vi "Wait For Key File.vi"(8 "error in":errorcluster, 11 "key file path":path) -> (0 "error out":errorcluster)   [LabVIEW 2020, in "Measurement Plugin Discovery V1.lvlib"]
uses:
  Measurement Plugin Discovery V1.lvlib
  Measurement Plugin Measurement Server/Helpers/Error Strings Global Internal.vi
  <vilib>/ErrorRing/Error Ring.xnode
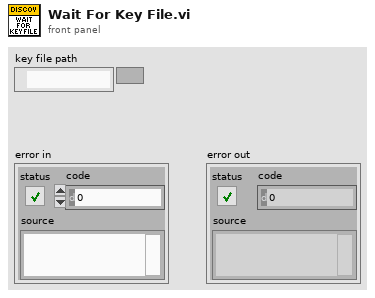
[diagram p1: front panel]
types:
  T1 = enum16{"open", "replace", "create", "open or create", "replace or create", "replace or create with confirmation"}
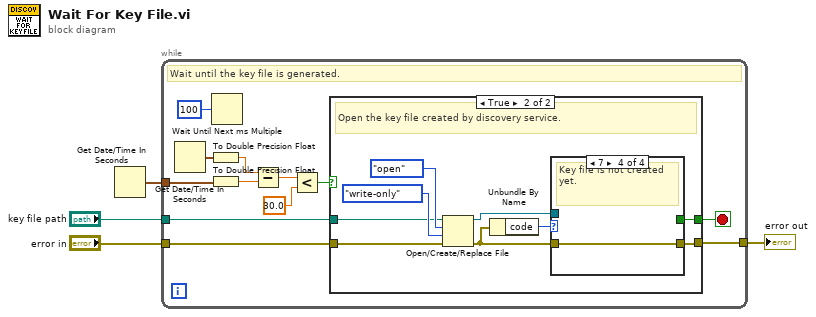
[diagram p0: block diagram]
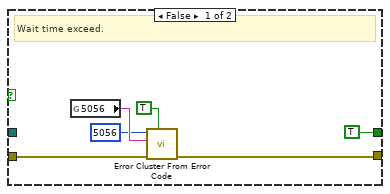
[diagram p2: hidden frame]
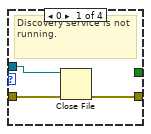
[diagram p3: hidden frame]
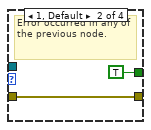
[diagram p4: hidden frame]
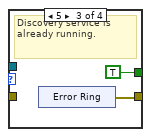
[diagram p5: hidden frame]
diagram:
  n1 = Get Date/Time In Seconds() -> (seconds since 1Jan1904=w1:timestamp)
  n2 = while {
    tunnel: "error in" -> [w13]
    tunnel: "key file path" -> [w14]
    tunnel: [w11] -> w3
    tunnel: w1 -> [w6]
    stop <- w12 stop-if-true
    # "Wait until the key file is generated."
    n3 = Get Date/Time In Seconds() -> (seconds since 1Jan1904=w7:timestamp)
    n4 = To Double Precision Float(number=w7) -> (double precision float=w8:dbl)
    n5 = To Double Precision Float(number=w6) -> (double precision float=w5:dbl)
    n6 = Wait Until Next ms Multiple(millisecond multiple=u32 100) -> ()  [unwired: 1 out]
    n7 = Subtract(x=w8, y=w5) -> (x-y=w9:dbl)
    n8 = Less?(x=w9, y=30.0) -> (x < y?=w16:bool)
    n9 = case shown="True" w16 {
      tunnel: w14 -> [_ w28]
      tunnel: w13 -> [w18 w29]
      tunnel: [TRUE w24] -> w12
      tunnel: [w17 w25] -> w11
      frame False {
        # "Wait time exceed."
        n10 = global read "Error Strings Global Internal.vi" "5056"() -> (w21:string)
        n11 = call <vilib>:"Error Cluster From Error Code.vi"("show call chain? (False)"=TRUE, "error in (no error)"=w18, "error message (\"\")"=w21, "error code (0)"=5056) -> ("error out"=w17:errorcluster)  [unwired: 5 in]
      }
      frame True {
        # "Open the key file created by discovery service."
        n12 = Open/Create/Replace File(file path (use dialog)=w28, error in=w29, operation (0:open)=T1."open", access (0:read/write)=enum16{"read/write", "read-only", "write-only"}."write-only") -> (refnum out=w23:refnum<file>, error out=w26:errorcluster)  [unwired: 2 in, 1 out]
        n13 = Unbundle By Name(w26) -> ("code"=w27:i32)
        n14 = case shown="7" w27 {
          tunnel: [w33 w36 w38 w40] -> w25
          tunnel: w26 -> [w34 w36 _ w40]
          tunnel: [_ TRUE TRUE _] -> w24
          tunnel: w23 -> [w32 _ _ _]
          frame 0 {
            # "Discovery service is not running."
            n15 = Close File(refnum=w32, error in=w34) -> (error out=w33:errorcluster)  [unwired: 1 out]
          }
          frame 1, Default {
            # "Error occurred in any of the previous node."
          }
          frame 5 {
            # "Discovery service is already running."
            n16 = xnode "Error Ring"() -> ("error out"=w38:errorcluster)
          }
          frame 7 {
            # "Key file is not created yet."
          }
        }
      }
    }
  }
  "error out" <- w3
